vi "Read Continuous Value (SubVI).vi"(8 "error in":errorcluster, 11 "VISA Refnum in":refnum<visa-resource-name>) -> (0 "error out":errorcluster, 1 "nombre":dbl, 3 "VISA Refnum out":refnum<visa-resource-name>, 5 "Data":string)   [LabVIEW 2017]
doc: "by Tanguy BOULARD"
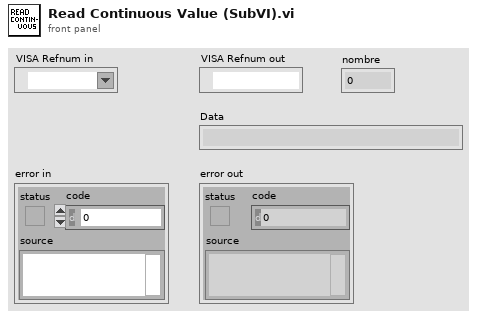
[diagram p1: front panel]
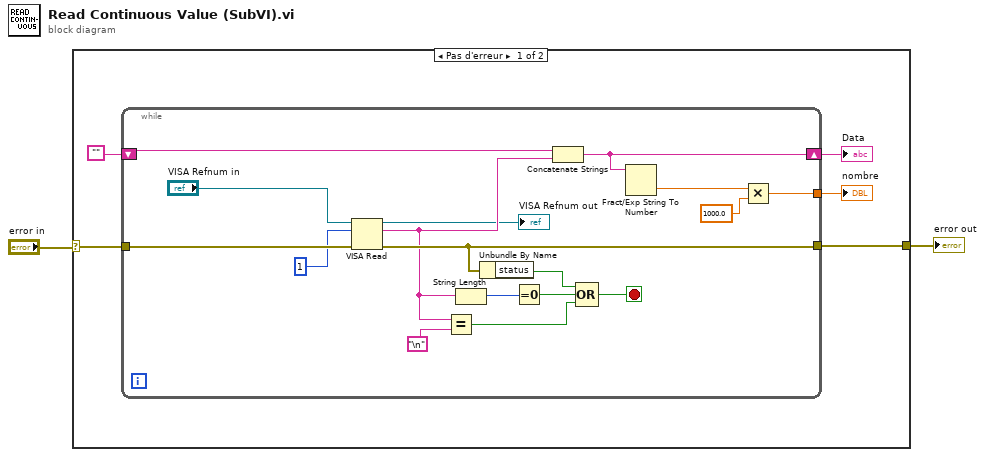
[diagram p0: block diagram]
diagram:
  n1 = case shown="Pas d'erreur" "error in" {
    selector: "error in" -> [w7 w25]
    tunnel: [w5 w25] -> w2
    frame No Error {
      n2 = while {
        shift-right: [w11] -> w4
        shift-left: "" -> [w24]
        tunnel: w7 -> [w23]
        tunnel: [w20] -> w5
        tunnel: [w8] -> w3
        stop <- w14 stop-if-true
        n3 = VISA Read(VISA resource name="VISA Refnum in", byte count=u32 1, error in (no error)=w23) -> (VISA resource name out=→"VISA Refnum out":refnum<visa-resource-name>, read buffer=w19:string, error out=w20:errorcluster)  [unwired: 1 out]
        n4 = Equal?(x=w19, y="\n") -> (x = y?=w15:bool)
        n5 = String Length(string=w19) -> (length=w18:i32)
        n6 = Unbundle By Name(w20) -> ("status"=w17:bool)
        n7 = Equal To 0?(x=w18) -> (x = 0?=w16:bool)
        n8 = Concatenate Strings(w24, w19) -> (w11:string)
        n9 = Compound Arithmetic op=OR(w17, w16, w15) -> (w14:bool)
        n10 = Fract/Exp String To Number(string=w11) -> (number=w9:dbl)  [unwired: 3 in, 1 out]
        n11 = Multiply(x=w9, y=1000.0) -> (x*y=w8:dbl)
      }
      "Data" <- w4
      "nombre" <- w3
    }
    frame Error {
    }
  }
  "error out" <- w2
